vi "set output range.vi"(9 "output range low (requested)":dbl, 10 "output range high (requested)":dbl, 11 "module editor in":refnum<data-value>) -> (0 "error out":errorcluster, 1 "output range low (real)":dbl, 2 "output range high (real)":dbl)   [LabVIEW 2013, in "My Awesome Control Modules editor node.lvclass"]
uses:
  My Awesome Control Modules editor node.lvclass
  <vilib>/NI/Tag Bus/tag/tag descriptor.lvclass
  <vilib>/NI/Tag Bus Data Framework/control module/configuration/control module configuration.lvclass
  <vilib>/NI/Tag Bus/tag/default value polymorphs/write default value Double.vi
  <vilib>/NI/Tag Bus Data Framework/control module/editor node/control module editor.lvclass
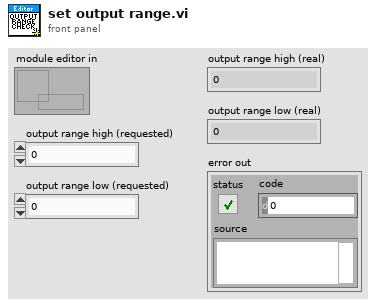
[diagram p1: front panel]
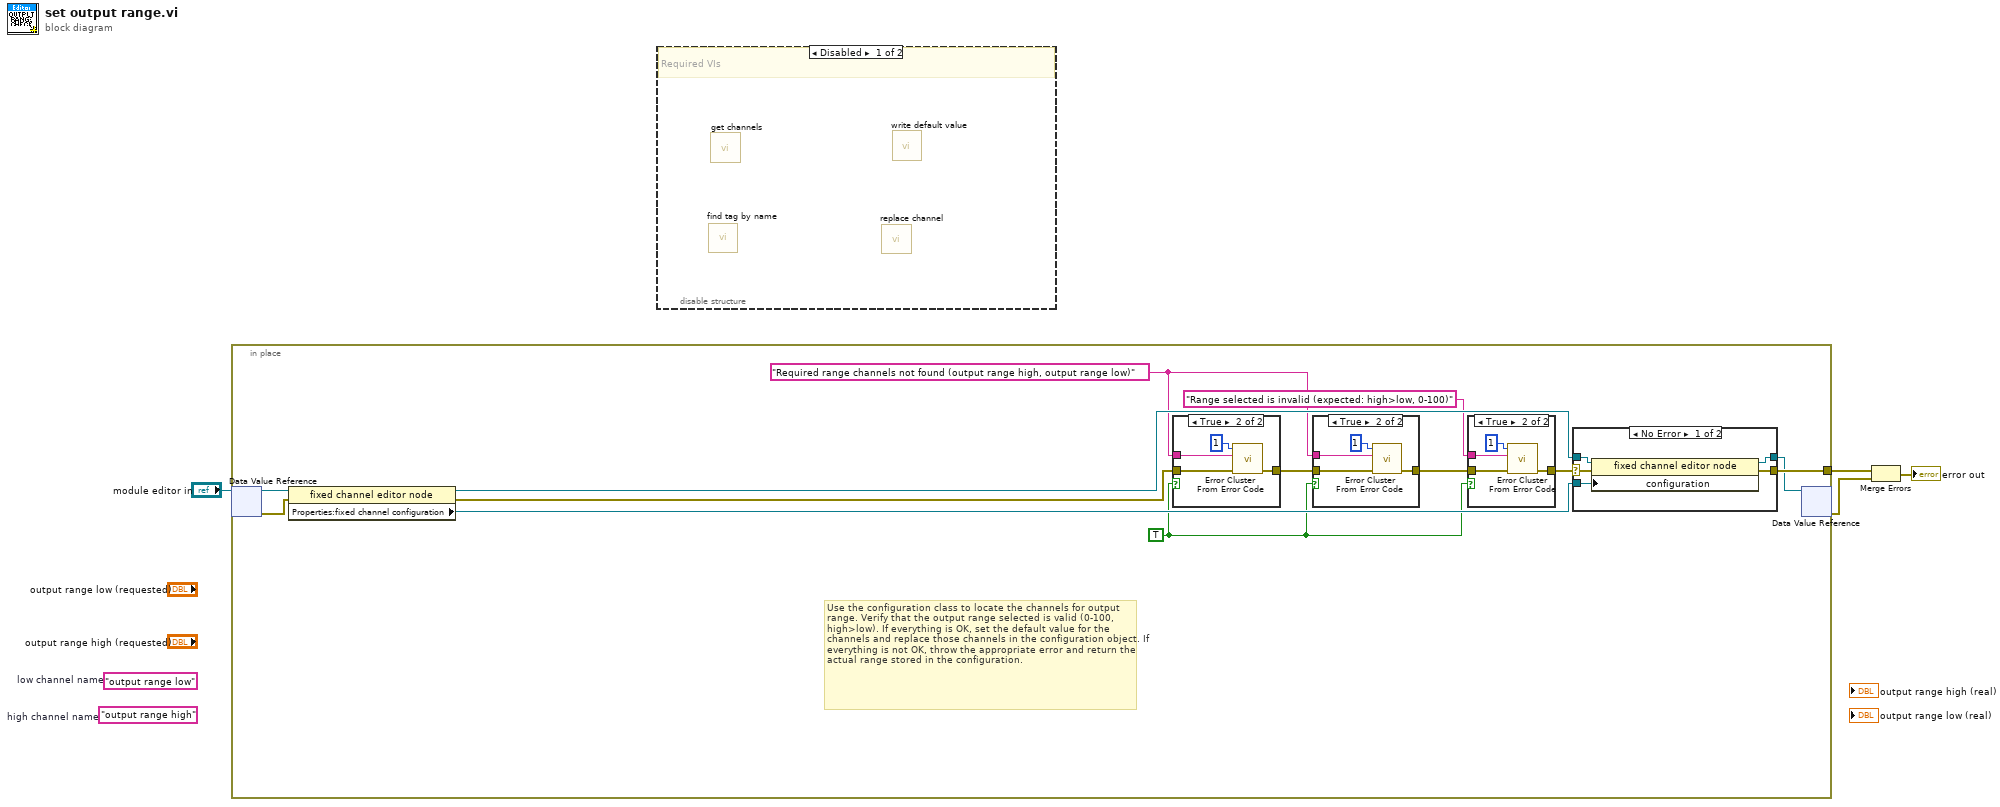
[diagram p0: block diagram]
diagram:
  (unwired) "output range low"  # low channel name
  (unwired) "output range high"  # high channel name
  n1 = in-place {
    in-place-border: [w14] -> w2
    w5 = TRUE
    w11 = "Required range channels not found (output range high, output range low)" ("error message (\"\")")
    # "Use the configuration class to locate the channels for output range. Verify that the output range selected is valid (0-100, high>low). If everything is OK, set the default value for the channels and replace those channels in the configuration object. If everything is not OK, throw the appropriate error and return the actual range stored in the configuration."
    n2 = in-place-dvr #1("module editor in") -> (w17:refnum<class "control module editor.lvclass">, w16:errorcluster)
    n3 = property class="fixed channel editor node"(reference=w17, error in=w16) -> (reference out=w15:refnum<class "control module editor.lvclass">, error out=w10:errorcluster, "Properties:fixed channel configuration"=w6:refnum<class "control module configuration.lvclass">)
    n4 = case shown="True" w5 {
      tunnel: w11 -> [_ w26]
      tunnel: [w23 w25] -> w9
      tunnel: w10 -> [w23 w24]
      frame False {
      }
      frame True {
        n5 = call <vilib>:"Error Cluster From Error Code.vi"("error in (no error)"=w24, "error message (\"\")"=w26, "error code (0)"=1) -> ("error out"=w25:errorcluster)  [unwired: 6 in]
      }
    }
    n6 = case shown="True" w5 {
      tunnel: w11 -> [_ w21]
      tunnel: [w18 w20] -> w8
      tunnel: w9 -> [w18 w19]
      frame False {
      }
      frame True {
        n7 = call <vilib>:"Error Cluster From Error Code.vi"("error in (no error)"=w19, "error message (\"\")"=w21, "error code (0)"=1) -> ("error out"=w20:errorcluster)  [unwired: 6 in]
      }
    }
    n8 = case shown="True" w5 {
      tunnel: "Range selected is invalid (expected: high>low, 0-100)" ("error message (\"\")") -> [_ w31]
      tunnel: [w28 w30] -> w7
      tunnel: w8 -> [w28 w29]
      frame False {
      }
      frame True {
        n9 = call <vilib>:"Error Cluster From Error Code.vi"("error in (no error)"=w29, "error message (\"\")"=w31, "error code (0)"=1) -> ("error out"=w30:errorcluster)  [unwired: 6 in]
      }
    }
    n10 = case shown="No Error" w7 {
      selector: w7 -> [w36 w39]
      tunnel: w15 -> [w37 w38]
      tunnel: [w35 w39] -> w14
      tunnel: [w34 w38] -> w13
      tunnel: w6 -> [w33 _]
      frame No Error {
        n11 = property class="fixed channel editor node"(reference=w37, error in=w36, "configuration"=w33) -> (reference out=w34:refnum<class "control module editor.lvclass">, error out=w35:errorcluster)
      }
      frame Error {
      }
    }
    n12 = in-place-dvr #1(w13) -> (w3:errorcluster)  [unwired: 1 out]
  }
  n13 = disable-structure shown="Disabled" {
    frame Disabled {
      # "Required VIs"
      n14 = call <vilib>:"find tag by name.vi"() -> ()  [unwired: 11 in, 1 out]
      n15 = call-dynamic "get channels.vi"() -> ()  [unwired: 10 in, 2 out]
      n16 = call <vilib>:"replace channel.vi"() -> ()  [unwired: 10 in, 2 out]
      n17 = call-poly <vilib>:"write default value.vi"() -> ()  [unwired: 10 in, 2 out]
    }
    frame Enabled {
    }
  }
  n18 = Merge Errors(w2, w3) -> (→"error out":errorcluster)
